vi "Digital Edge Trigger.vi"(8 "error in":errorcluster, 10 "Source":string, 11 "4300 in":refnum<class "4300.lvclass">) -> (0 "error out":errorcluster, 3 "4300 out":refnum<class "4300.lvclass">)   [LabVIEW 2019, in "4300.lvlib" / "4300.lvclass"]
uses:
  Library/4300.lvclass
  C:/Users/Public/Documents/Development/builds/Instruments/AnalogInput.lvlibp/Library/AnalogInput.lvclass
  Library/4300.lvclass/4300.ctl
  builds/Instruments/AnalogInput.lvlibp/Accessors/Triggering/Read Trigger Settings.vi
  <vilib>/DAQmx/configure/trigger.llb/DAQmx Reference Trigger (Digital Edge).vi
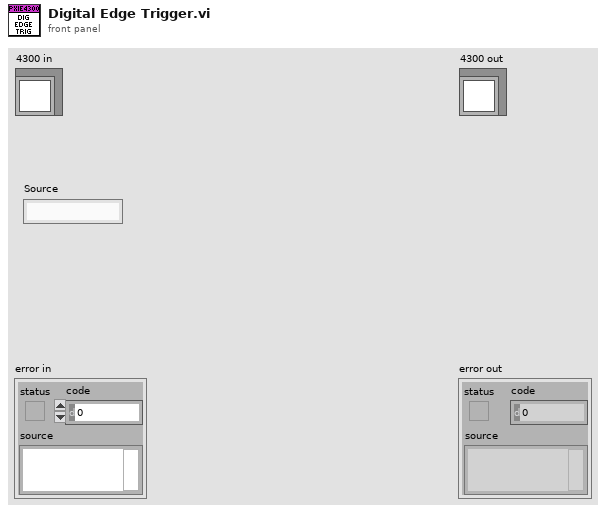
[diagram p1: front panel]
types:
  T1 = typedef "AnalogInput.lvlibp/AnalogInput.lvclass/User Trigger Settings.ctl" = cluster{"Timeout":dbl, "Level":dbl, "Slope":T2, "samples per channel":i32, "Sample Rate (10k)":dbl, "pretrigger samples":u32}
  T2 = typedef "AnalogInput.lvlibp/AnalogInput.lvclass/Trigger_Slope.ctl" = enum16{"Rising", "Falling"}
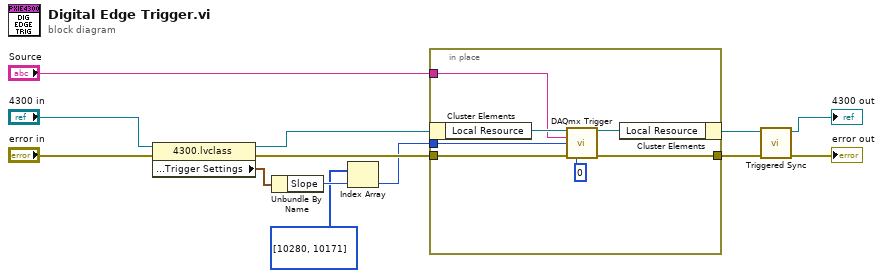
[diagram p0: block diagram]
diagram:
  w10 = i32[] [10280, 10171] items=["Rising"=10280, "Falling"=10171]
  n1 = property class="4300.lvclass"(reference="4300 in", error in="error in") -> (reference out=w8:refnum<class "4300.lvclass">, error out=w13:errorcluster, "Accessors:Triggering:Trigger Settings"=w12:T1)
  n2 = Unbundle By Name(w12) -> ("Slope"=w11:T2)
  n3 = Index Array(array=w10, index=w11) -> (element=w9:i32)
  n4 = in-place {
    in-place-border: w13 -> [w20]
    in-place-border: "Source" -> [w14]
    in-place-border: [w18] -> w7
    in-place-border: w9 -> [w17]
    n5 = in-place-cluster #1(w8) -> ("Local Resource"=w16:refnum<k21>)
    n6 = call-poly <vilib>:"DAQmx Trigger.vi"("task/channels in"=w16, "source"=w14, "edge"=w17, "error in"=w20, "pretrigger samples per channel"=u32 0) -> ("task out"=w15:refnum<k21>, "error out"=w18:errorcluster)  [unwired: 9 in]
    n7 = in-place-cluster #1("Local Resource"=w15) -> (w2:refnum<class "4300.lvclass">)
  }
  n8 = call "Triggered Sync.vi"("error in"=w7, "4300 in"=w2) -> ("error out"=→"error out":errorcluster, "4300 out"=→"4300 out":refnum<class "4300.lvclass">)  [unwired: 8 in]
